vi "devide.vi"(10 "String 2":string, 11 "String":string) -> (3 "String 3":string)   [LabVIEW 2025]
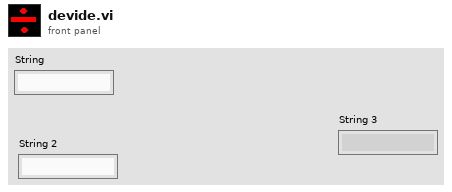
[diagram p1: front panel]
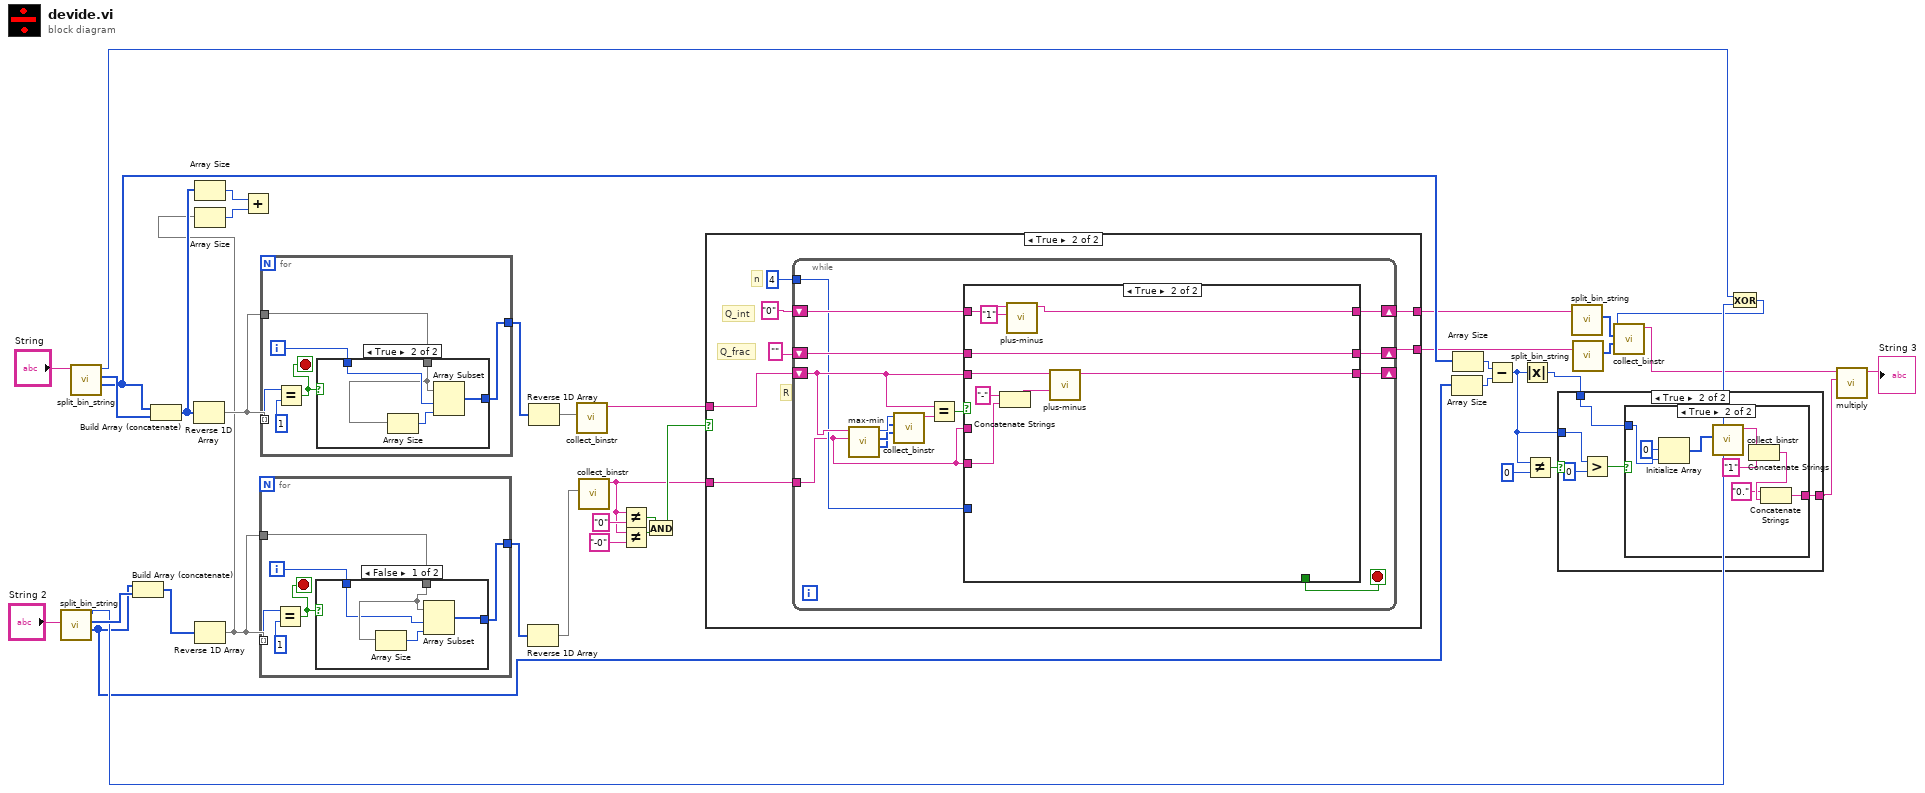
[diagram p0: block diagram]
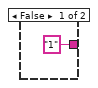
[diagram p2: hidden frame]
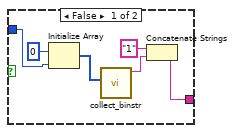
[diagram p3: hidden frame]
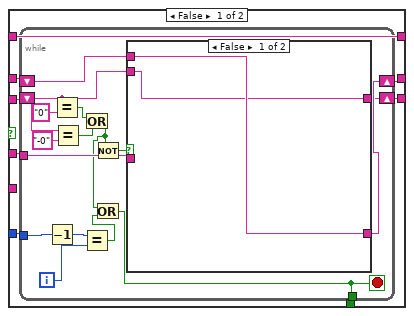
[diagram p5: hidden frame]
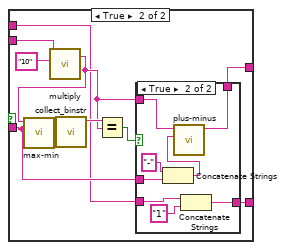
[diagram p6: hidden frame]
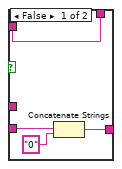
[diagram p7: hidden frame]
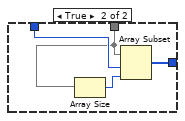
[diagram p8: hidden frame]
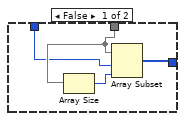
[diagram p9: hidden frame]
diagram:
  n1 = call "split_bin_string.vi"("String"="String 2") -> ("Fraction"=w15:u8[], "Integer"=w36:u8[], "Sign"=w24:u8)  [unwired: 8 in]
  n2 = call "split_bin_string.vi"("String"="String") -> ("Fraction"=w16:u8[], "Integer"=w37:u8[], "Sign"=w25:u8)  [unwired: 8 in]
  n3 = Build Array (concatenate)(w15, w36) -> (w31:u8[])
  n4 = Build Array (concatenate)(w16, w37) -> (w29:u8[])
  n5 = Reverse 1D Array(array=w29) -> (reversed array=w35:u8[])
  n6 = Array Size(array=w29) -> (size(s)=w26:i32)
  n7 = Reverse 1D Array(array=w31) -> (reversed array=w28:u8[])
  n8 = Array Size(array=w28) -> (size(s)=w27:i32)
  n9 = Add(x=w26, y=w27) -> ()  [unwired: 1 out]
  n10 = for {
    tunnel: w28 -> [w45] mode=indexing
    tunnel: w28 -> [w41]
    tunnel: [w40] -> w32
    i -> [w42]
    stop <- w43 stop-if-true
    n11 = Equal?(x=w45, y=u8 1) -> (x = y?=w43:bool)
    n12 = case shown="False" w43 {
      tunnel: w42 -> [w46 w53]
      tunnel: w41 -> [w49 w52]
      tunnel: [w47 w50] -> w40
      frame False {
        n13 = Array Size(array=w49) -> (size(s)=w48:i32)
        n14 = Array Subset(array=w49, index=w46, length=w48) -> (w47:u8[])
      }
      frame True {
        n15 = Array Size(array=w52) -> (size(s)=w51:i32)
        n16 = Array Subset(array=w52, index=w53, length=w51) -> (w50:u8[])
      }
    }
  }
  n17 = for {
    tunnel: w35 -> [w59] mode=indexing
    tunnel: w35 -> [w55]
    tunnel: [w54] -> w34
    i -> [w56]
    stop <- w57 stop-if-true
    n18 = Equal?(x=w59, y=u8 1) -> (x = y?=w57:bool)
    n19 = case shown="True" w57 {
      tunnel: w56 -> [w60 w67]
      tunnel: w55 -> [w63 w66]
      tunnel: [w61 w64] -> w54
      frame False {
        n20 = Array Size(array=w63) -> (size(s)=w62:i32)
        n21 = Array Subset(array=w63, index=w60, length=w62) -> (w61:u8[])
      }
      frame True {
        n22 = Array Size(array=w66) -> (size(s)=w65:i32)
        n23 = Array Subset(array=w66, index=w67, length=w65) -> (w64:u8[])
      }
    }
  }
  n24 = Reverse 1D Array(array=w32) -> (reversed array=w30:u8[])
  n25 = Reverse 1D Array(array=w34) -> (reversed array=w33:u8[])
  n26 = call "collect_binstr.vi"("Integer"=w33) -> ("String"=w23:string)  [unwired: 10 in]
  n27 = call "collect_binstr.vi"("Integer"=w30) -> ("String"=w17:string)  [unwired: 10 in]
  n28 = Not Equal?(x=w17, y="0") -> (x != y?=w21:bool)
  n29 = Not Equal?(x=w17, y="-0") -> (x != y?=w20:bool)
  n30 = And(x=w21, y=w20) -> (x .and. y?=w22:bool)
  n31 = case shown="True" w22 {
    tunnel: w23 -> [_ w72]
    tunnel: w17 -> [_ w70]
    tunnel: [_ w69] -> w9
    tunnel: [_ w68] -> w12
    frame False {
    }
    frame True {
      # "n"
      # "R"
      # "Q_frac"
      # "Q_int"
      n32 = while {
        shift-right: [w75] -> _
        shift-left: w72 -> [w81]
        tunnel: 4 -> [w78]
        tunnel: w70 -> [w77]
        shift-right: [w82] -> w69
        shift-left: "0" -> [w83]
        shift-right: [w79] -> w68
        shift-left: "" -> [w80]
        stop <- w76 stop-if-true
        n33 = call "max-min.vi"("String 2"=w77, "String"=w81) -> ("Fraction"=w86:u8[], "Integer"=w87:u8[], "Sign"=w88:u8)  [unwired: 4 in, 3 out]
        n34 = call "collect_binstr.vi"("Fraction"=w86, "Integer"=w87, "Sign"=w88) -> ("String"=w85:string)  [unwired: 8 in]
        n35 = Equal?(x=w81, y=w85) -> (x = y?=w84:bool)
        n36 = case shown="True" w84 {
          tunnel: w81 -> [w96 w147]
          tunnel: w77 -> [_ w140]
          tunnel: [w89 w146] -> w75
          tunnel: w83 -> [w91 w145]
          tunnel: [w91 w143] -> w82
          tunnel: w80 -> [w94 w142]
          tunnel: [w90 w142] -> w79
          tunnel: w78 -> [w93 _]
          tunnel: w77 -> [w95 _]
          tunnel: [w92 _] -> w76
          frame False {
            n37 = while {
              tunnel: w95 -> [w107]
              tunnel: w93 -> [w98]
              tunnel: [w102] -> w92
              shift-right: [w100] -> w90
              shift-left: w94 -> [w106]
              shift-right: [w97] -> w89
              shift-left: w96 -> [w108]
              i -> [w101]
              stop <- w102 stop-if-true
              n38 = Decrement(x=w98) -> (x-1=w99:i32)
              n39 = Equal?(x=w108, y="0") -> (x = y?=w110:bool)
              n40 = Equal?(x=w108, y="-0") -> (x = y?=w109:bool)
              n41 = Or(x=w110, y=w109) -> (x .or. y?=w103:bool)
              n42 = Equal?(x=w99, y=w101) -> (x = y?=w104:bool)
              n43 = Not(x=w103) -> (.not. x?=w105:bool)
              n44 = Or(x=w103, y=w104) -> (x .or. y?=w102:bool)
              n45 = case shown="False" w105 {
                tunnel: w108 -> [w113 w126]
                tunnel: w107 -> [_ w118]
                tunnel: w106 -> [w114 w117]
                tunnel: [w114 w116] -> w100
                tunnel: [w113 w115] -> w97
                frame False {
                }
                frame True {
                  n46 = call "multiply.vi"("String 2"="10", "String"=w126) -> ("String 3"=w119:string)  [unwired: 9 in]
                  n47 = call "max-min.vi"("String 2"=w118, "String"=w119) -> ("Fraction"=w122:u8[], "Integer"=w123:u8[], "Sign"=w124:u8)  [unwired: 4 in, 3 out]
                  n48 = call "collect_binstr.vi"("Fraction"=w122, "Integer"=w123, "Sign"=w124) -> ("String"=w121:string)  [unwired: 8 in]
                  n49 = Equal?(x=w121, y=w119) -> (x = y?=w120:bool)
                  n50 = case shown="True" w120 {
                    tunnel: w119 -> [w128 w138]
                    tunnel: w118 -> [_ w135]
                    tunnel: [w128 w134] -> w115
                    tunnel: w117 -> [w127 w132]
                    tunnel: [w129 w131] -> w116
                    frame False {
                      n51 = Concatenate Strings(w127, "0" ("string")) -> (w129:string)
                    }
                    frame True {
                      n52 = Concatenate Strings("-" ("string"), w135) -> (w137:string)
                      n53 = call "plus-minus.vi"("String 2"=w137, "String"=w138) -> ("String 3"=w134:string)  [unwired: 9 in]
                      n54 = Concatenate Strings(w132, "1" ("string")) -> (w131:string)
                    }
                  }
                }
              }
            }
          }
          frame True {
            n55 = Concatenate Strings("-" ("string"), w140) -> (w139:string)
            n56 = call "plus-minus.vi"("String 2"="1", "String"=w145) -> ("String 3"=w143:string)  [unwired: 9 in]
            n57 = call "plus-minus.vi"("String 2"=w139, "String"=w147) -> ("String 3"=w146:string)  [unwired: 9 in]
          }
        }
      }
    }
  }
  n58 = Array Size(array=w15) -> (size(s)=w13:i32)
  n59 = Array Size(array=w16) -> (size(s)=w14:i32)
  n60 = Subtract(x=w14, y=w13) -> (x-y=w3:i32)
  n61 = Absolute Value(x=w3) -> (abs(x)=w2:i32)
  n62 = Not Equal?(x=w3, y=0) -> (x != y?=w4:bool)
  n63 = case shown="True" w4 {
    tunnel: w3 -> [_ w153]
    tunnel: w2 -> [_ w150]
    tunnel: ["1" w149] -> w1
    frame False {
    }
    frame True {
      n64 = Greater?(x=w153, y=0) -> (0:w151:bool)
      n65 = case shown="True" w151 {
        tunnel: w150 -> [w158 w166]
        tunnel: [w156 w162] -> w149
        frame False {
          n66 = Initialize Array(u8 0 ("element"), w158) -> (w155:u8[])
          n67 = call "collect_binstr.vi"("Integer"=w155) -> ("String"=w154:string)  [unwired: 10 in]
          n68 = Concatenate Strings("1" ("string"), w154) -> (w156:string)
        }
        frame True {
          n69 = Initialize Array(u8 0 ("element"), w166) -> (w160:u8[])
          n70 = call "collect_binstr.vi"("Integer"=w160) -> ("String"=w161:string)  [unwired: 10 in]
          n71 = Concatenate Strings(w161, "1" ("string")) -> (w164:string)
          n72 = Concatenate Strings("0." ("string"), w164) -> (w162:string)
        }
      }
    }
  }
  n73 = call "split_bin_string.vi"("String"=w9) -> ("Integer"=w11:u8[])  [unwired: 8 in, 2 out]
  n74 = call "split_bin_string.vi"("String"=w12) -> ("Integer"=w10:u8[])  [unwired: 8 in, 2 out]
  n75 = Exclusive Or(1:w24, 2:w25) -> (0:w6:u8)
  n76 = call "collect_binstr.vi"("Fraction"=w10, "Integer"=w11, "Sign"=w6) -> ("String"=w8:string)  [unwired: 8 in]
  n77 = call "multiply.vi"("String 2"=w1, "String"=w8) -> ("String 3"=→"String 3":string)  [unwired: 9 in]
